vi "Collapse Mode Array SLM2.vi"(2 "Action":u16(ring) items=["Read", "Initialize"], 7 "mode array":dbl[][][](array[numeric])) -> (8 "collapsed mode array":dbl[][](array[numeric]))   [LabVIEW 2014]
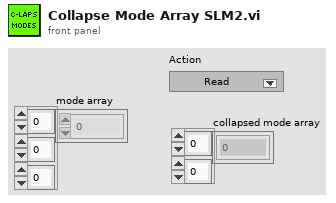
[diagram p1: front panel]
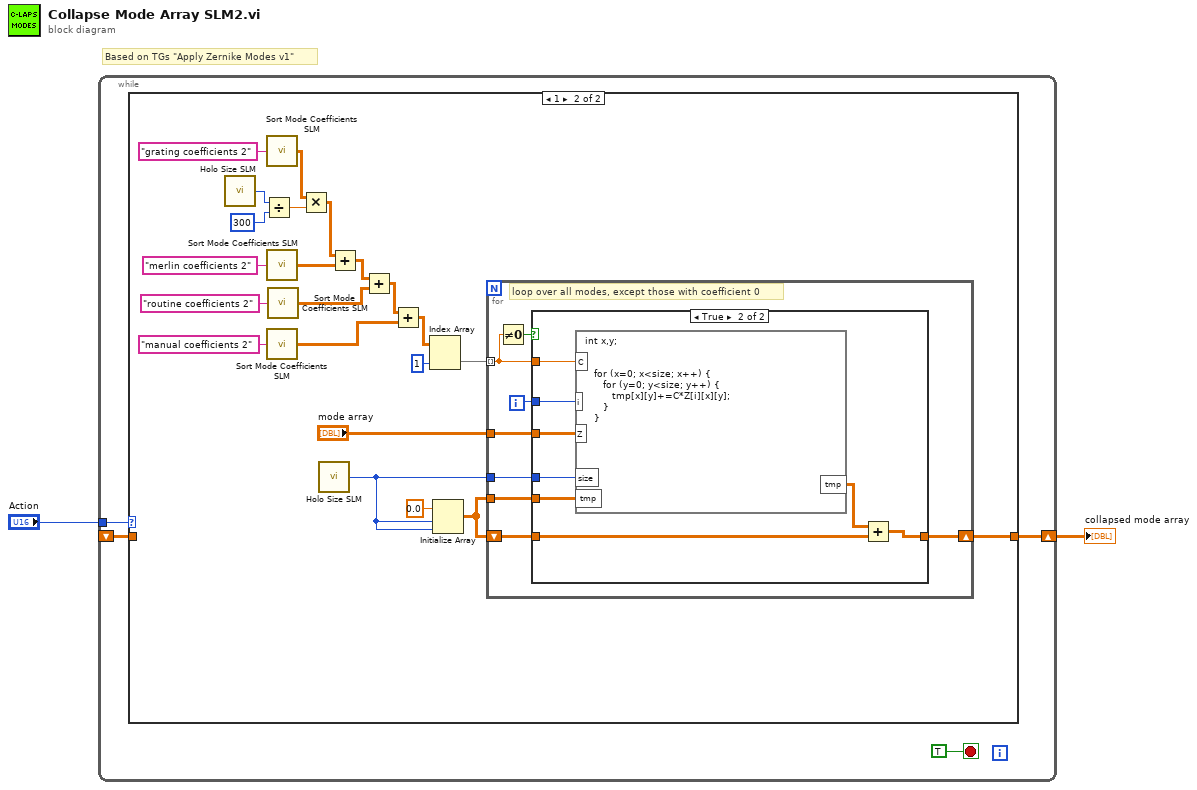
[diagram p0: block diagram]
diagram:
  # "Based on TGs \"Apply Zernike Modes v1\""
  n1 = while {
    shift-right: [w3] -> w1
    shift-left: _ -> [w4]
    tunnel: "Action" -> [w5]
    stop <- TRUE stop-if-true
    n2 = case shown="1" w5 {
      tunnel: w4 -> [w7 _]
      tunnel: [w7 w24] -> w3
      frame 0, Default {
      }
      frame 1 {
        n3 = call "Holo Size SLM.vi"() -> ("data"=w12:i32)  [unwired: 15 in]
        n4 = Divide(x=w12, y=300) -> (x/y=w9:dbl)
        n5 = call "Sort Mode Coefficients SLM.vi"("coefficient source"="grating coefficients 2") -> ("coefficient list"=w10:dbl[][])  [unwired: 14 in]
        n6 = call "Sort Mode Coefficients SLM.vi"("coefficient source"="merlin coefficients 2") -> ("coefficient list"=w15:dbl[][])  [unwired: 14 in]
        n7 = call "Sort Mode Coefficients SLM.vi"("coefficient source"="manual coefficients 2") -> ("coefficient list"=w19:dbl[][])  [unwired: 14 in]
        n8 = call "Sort Mode Coefficients SLM.vi"("coefficient source"="routine coefficients 2") -> ("coefficient list"=w20:dbl[][])  [unwired: 14 in]
        n9 = Multiply(x=w10, y=w9) -> (x*y=w8:dbl[][])
        n10 = call "Holo Size SLM.vi"() -> ("data"=w29:i32)  [unwired: 15 in]
        n11 = Add(x=w8, y=w15) -> (x+y=w14:dbl[][])
        n12 = Add(x=w14, y=w20) -> (x+y=w18:dbl[][])
        n13 = Add(x=w18, y=w19) -> (x+y=w17:dbl[][])
        n14 = Index Array(array=w17, index (col)=1 ("index")) -> (element=w26:dbl[])  [unwired: 1 in]
        n15 = Initialize Array(0.0 ("element"), w29, w29) -> (w28:dbl[][])
        n16 = for {
          shift-right: [w30] -> w24
          shift-left: w28 -> [w31]
          tunnel: "mode array" -> [w34]
          tunnel: w29 -> [w37]
          tunnel: w26 -> [w33] mode=indexing
          tunnel: w28 -> [w36]
          i -> [w35]
          # "loop over all modes, except those with coefficient 0"
          n17 = Not Equal To 0?(x=w33) -> (x != 0?=w32:bool)
          n18 = case shown="True" w32 {
            tunnel: w37 -> [_ w46]
            tunnel: w36 -> [_ w45]
            tunnel: w33 -> [_ w44]
            tunnel: w35 -> [_ w43]
            tunnel: w34 -> [_ w42]
            tunnel: w31 -> [w38 w40]
            tunnel: [w38 w39] -> w30
            frame False {
            }
            frame True {
              n19 = formula code="int x,y;\n\n\n   for (x=0; x<size; x++) {\n      for (y=0; y<size; y++) {\n         tmp[x][y]+=C*Z[i][x][y];\n      }\n   }"("C"=w44, "size"=w46, "tmp"=w45, "i"=w43, "Z"=w42) -> ("tmp"=w41:dbl[][])
              n20 = Add(x=w41, y=w40) -> (x+y=w39:dbl[][])
            }
          }
        }
      }
    }
  }
  "collapsed mode array" <- w1
